vi "giveStim.vi"(8 "error in (no error)":errorcluster, 10 "data":bool[](array[boolean]), 11 "Stim in":refnum<class "Stim.lvclass">) -> (0 "error out":errorcluster, 3 "Stim out":refnum<class "Stim.lvclass">)   [LabVIEW 2014, in "Stim.lvclass"]
uses:
  Stim.lvclass
  Stim.lvclass/Stim.ctl
  <vilib>/DAQmx/write.llb/DAQmx Write.vi
  <vilib>/DAQmx/write.llb/DAQmx Write (Digital 1D Bool NChan 1Samp 1Line).vi
  <vilib>/DAQmx/miscellaneous.llb/DAQmx Fill In Error Info.vi
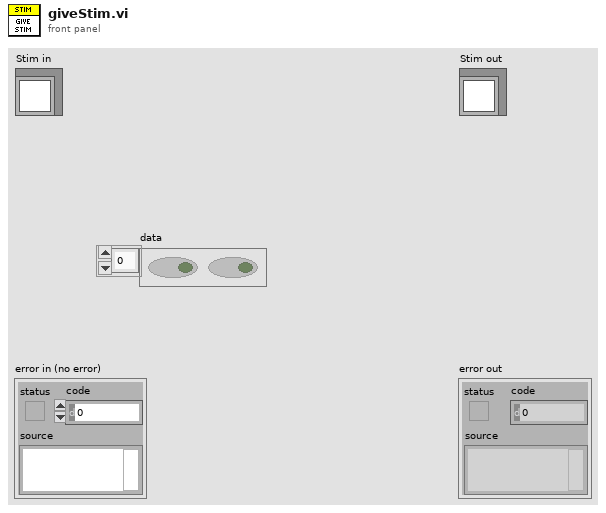
[diagram p1: front panel]
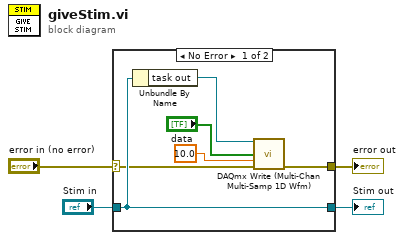
[diagram p0: block diagram]
diagram:
  n1 = case shown="No Error" "error in (no error)" {
    selector: "error in (no error)" -> [w7 w12]
    tunnel: [w6 w12] -> w2
    tunnel: [w9 w11] -> w1
    tunnel: "Stim in" -> [w9 w11]
    frame No Error {
      n2 = Unbundle By Name(w9) -> ("task out"=w8:refnum<k21>)
      n3 = call-poly "DAQmx Write (Multi-Chan Multi-Samp 1D Wfm).vi"("task/channels in"=w8, "data"="data", "timeout"=10.0, "error in"=w7) -> ("error out"=w6:errorcluster)  [unwired: 9 in, 2 out]
    }
    frame Error {
    }
  }
  "error out" <- w2
  "Stim out" <- w1
